vi "showLine.vi"(7 "mirror":bool, 10 "location":T1, 11 "colors":u32[](array[numeric])) -> (0 "error out":errorcluster)   [LabVIEW 2014]
uses:
  location.ctl
  pixxelAction.ctl
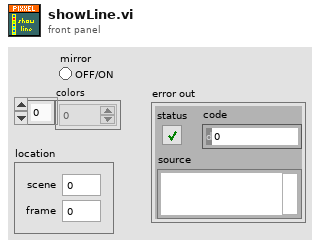
[diagram p1: front panel]
types:
  T1 = typedef "location.ctl" = cluster{"scene":u8, "frame":u8}
  T2 = typedef "pixxelAction.ctl" = enum16{"init", "watchdog", "setColor", "showSceneFrame", "black", "play", "close", "uploadProg", "startProg", "pauseProg", "continueProg", "jumpTo", "setIP", "setGW"}
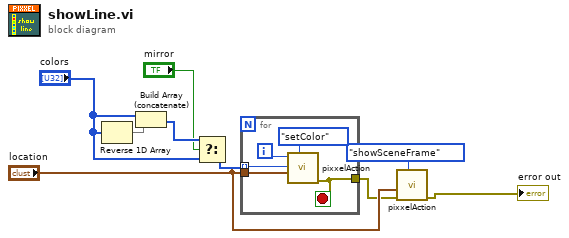
[diagram p0: block diagram]
diagram:
  n1 = Reverse 1D Array(array="colors") -> (reversed array=w5:u32[])
  n2 = Build Array (concatenate)("colors", w5) -> (w4:u32[])
  n3 = Select(t=w4, s="mirror", f="colors") -> (s? t:f=w3:u32[])
  n4 = for {
    tunnel: [w11] -> w7
    tunnel: w3 -> [w14] mode=indexing
    tunnel: "location" -> [w10]
    i -> [w12]
    stop <- w11 stop-if-true
    n5 = call "pixxelAction.vi"("PIXXELaction"=pixxelAction."setColor", "location"=w10, "color"=w14, "Pixel-nummer"=w12) -> ("error out"=w11:errorcluster)  [unwired: 7 in]
  }
  n6 = call "pixxelAction.vi"("PIXXELaction"=pixxelAction."showSceneFrame", "error in (no error)"=w7, "location"="location") -> ("error out"=→"error out":errorcluster)  [unwired: 8 in]
